vi "Destroy Suggestion Box.vi"(0 "Suggestion Box in":refnum<class "Suggestion Box.lvclass">, 11 "error in (no error)":errorcluster) -> (4 "Suggestion Box out":refnum<class "Suggestion Box.lvclass">, 15 "error out":errorcluster)   [LabVIEW 2016, in "Suggestion Box.lvclass"]
doc: "Stops and cleans up the Suggestion Box panel.\n--------------------\nCopyright (c) 2019 Analog Devices, Inc. All rights reserved.\n\nRedistribution and use in source and binary forms, with or without modification,\nare permitted provided that the following conditions are met:\n - Redistributions of source code must retain the above copyright notice, this\n list of conditions and the following disclaimer.\n - Redistributions in binary form must reproduce the above copyright notice,\n this list of conditions and the following disclaimer in the documentation\n and/or other materials provided with the distribution.\n - Modified versions of the software must be conspicuously marked as such.\n - This software is licensed solely and exclusively for use with\n processors/products manufactured by or for Analog Devices, Inc.\n - This software may not be combined or merged with other code in any manner\n that would cause the software to become subject to terms and conditions\n which differ from those listed here.\n - Neither the name of Analog Devices, Inc. nor the names of its contributors\n may be used to endorse or promote products derived from this software\n without specific prior written permission.\n - The use of this software may or may not infringe the patent rights of one or\n more patent holders. This license does not release you from the requirement\n that you obtain separate licenses from these patent holders to use this\n software.\n\nTHIS SOFTWARE IS PROVIDED BY ANALOG DEVICES, INC. AND CONTRIBUTORS \"AS IS\" AND\nANY EXPRESS OR IMPLIED WARRANTIES, INCLUDING, BUT NOT LIMITED TO,\nNON-INFRINGEMENT, TITLE, MERCHANTABILITY AND FITNESS FOR A PARTICULAR PURPOSE\nARE DISCLAIMED. IN NO EVENT SHALL ANALOG DEVICES, INC. OR CONTRIBUTORS BE LIABLE\nFOR ANY DIRECT, INDIRECT, INCIDENTAL, SPECIAL, EXEMPLARY, PUNITIVE OR\nCONSEQUENTIAL DAMAGES (INCLUDING, BUT NOT LIMITED TO, DAMAGES ARISING OUT OF\nCLAIMS OF INTELLECTUAL PROPERTY RIGHTS INFRINGEMENT; PROCUREMENT OF SUBSTITUTE\nGOODS OR SERVICES; LOSS OF USE, DATA, OR PROFITS; OR BUSINESS INTERRUPTION)\nHOWEVER CAUSED AND ON ANY THEORY OF LIABILITY, WHETHER IN CONTRACT, STRICT\nLIABILITY, OR TORT (INCLUDING NEGLIGENCE OR OTHERWISE) ARISING IN ANY WAY OUT OF\nTHE USE OF THIS SOFTWARE, EVEN IF ADVISED OF THE POSSIBILITY OF SUCH DAMAGE.\n\n2019-01-10-7CBSD SLA"
uses:
  Suggestion Box.lvclass
  Suggestion Box.lvclass/Suggestion Box.ctl
panel:
  # "Copyright (c) 2019 Analog Devices, Inc.  All rights reserved.\n\nRedistribution and use in source and binary forms, with or without modification,\nare permitted provided that the following conditions are met:\n  - Redistributions of source code must retain the above copyright notice, this\n    list of conditions and the following disclaimer.\n  - Redistributions in binary form must reproduce the above copyright notice,\n    this list of conditions and the following disclaimer in the documentation\n    and/or other materials provided with the distribution.\n  - Modified versions of the software must be conspicuously marked as such.\n  - This software is licensed solely and exclusively for use with\n    processors/products manufactured by or for Analog Devices, Inc.\n  - This software may not be combined or merged with other code in any manner\n    that would cause the software to become subject to terms and conditions\n    which differ from those listed here.\n  - Neither the name of Analog Devices, Inc. nor the names of its contributors\n    may be used to endorse or promote products derived from this software\n    without specific prior written permission.\n  - The use of this software may or may not infringe the patent rights of one or\n    more patent holders.  This license does not release you from the requirement\n    that you obtain separate licenses from these patent holders to use this\n    software.\n\nTHIS SOFTWARE IS PROVIDED BY ANALOG DEVICES, INC. AND CONTRIBUTORS \"AS IS\" AND\nANY EXPRESS OR IMPLIED WARRANTIES, INCLUDING, BUT NOT LIMITED TO,\nNON-INFRINGEMENT, TITLE, MERCHANTABILITY AND FITNESS FOR A PARTICULAR PURPOSE\nARE DISCLAIMED. IN NO EVENT SHALL ANALOG DEVICES, INC. OR CONTRIBUTORS BE LIABLE\nFOR ANY DIRECT, INDIRECT, INCIDENTAL, SPECIAL, EXEMPLARY, PUNITIVE OR\nCONSEQUENTIAL DAMAGES (INCLUDING, BUT NOT LIMITED TO, DAMAGES ARISING OUT OF\nCLAIMS OF INTELLECTUAL PROPERTY RIGHTS INFRINGEMENT; PROCUREMENT OF SUBSTITUTE\nGOODS OR SERVICES; LOSS OF USE, DATA, OR PROFITS; OR BUSINESS INTERRUPTION)\nHOWEVER CAUSED AND ON ANY THEORY OF LIABILITY, WHETHER IN CONTRACT, STRICT\nLIABILITY, OR TORT (INCLUDING NEGLIGENCE OR OTHERWISE) ARISING IN ANY WAY OUT OF\nTHE USE OF THIS SOFTWARE, EVEN IF ADVISED OF THE POSSIBILITY OF SUCH DAMAGE.\n\n2019-01-10-7CBSD SLA"
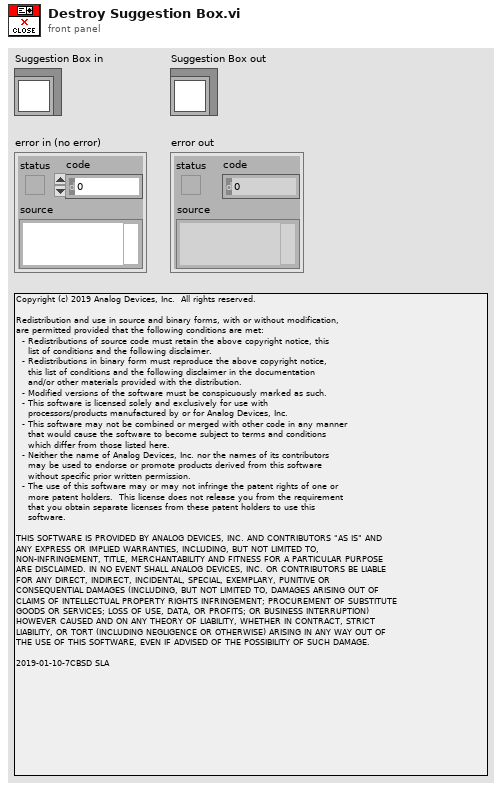
[diagram p1: front panel]
types:
  T1 = typedef "Rendezvous RefNum" = refnum<k1>
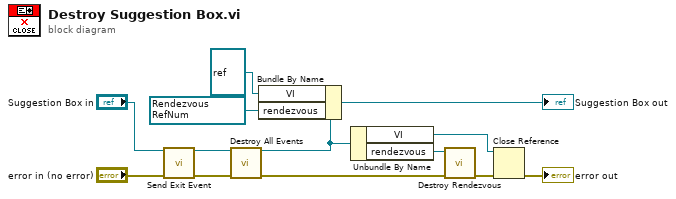
[diagram p0: block diagram]
diagram:
  w4 = T1 refnum items=["rendezvous"] ("rendezvous")
  n1 = call "Send Exit Event.vi"("Suggestion Box in"="Suggestion Box in", "error in (no error)"="error in (no error)") -> ("Suggestion Box out"=w1:refnum<class "Suggestion Box.lvclass">, "error out"=w3:errorcluster)  [unwired: 12 in]
  n2 = call "Destroy All Events.vi"("Suggestion Box in"=w1, "error in (no error)"=w3) -> ("Suggestion Box out"=w5:refnum<class "Suggestion Box.lvclass">, "error out"=w10:errorcluster)  [unwired: 12 in]
  n3 = Bundle By Name(cluster=w5, "VI"=refnum<vi> refnum ("VI Refnum"), "rendezvous"=w4) -> (→"Suggestion Box out":refnum<class "Suggestion Box.lvclass">)
  n4 = Unbundle By Name(w5) -> ("VI"=w12:refnum<vi>, "rendezvous"=w11:T1)
  n5 = call <vilib>:"Destroy Rendezvous.vi"("error in (no error)"=w10, "rendezvous"=w11) -> ("error out"=w8:errorcluster)  [unwired: 4 in, 1 out]
  n6 = Close Reference(reference=w12, error in (no error)=w8) -> (error out=→"error out":errorcluster)
